vi "GISStatus_XML_Read.vi"(8 "error in (no error)":errorcluster, 11 "XML String":string="<?xml version=\"1.0\" encoding=\"utf-8\"?>\n<PrintHeadStatusXML>    \n\t<PrintManager Name=\"Print Manager\" NodeName=\"PrintManager\" Type=\"1\">        \n\t\t<PrintLineManager Name=\"Print Line Manager\" NodeName=\"PrintLineManager\" Type=\"2\">            \n\t\t\t<PrintManagerBoard Name=\"PMB-KM\" NodeName=\"PrintManagerBoard\" Type=\"3\">                \n\t\t\t\t<H Name=\"HIB1-KM1024i\" NodeName=\"HIB\" Type=\"4\" Handle=\"000001B03748C210\" HeadEnabled=\"True\" SpitEnabled=\"True\" Status=\"16\" HeaterEnabled=\"True\" TargetTemperature=\"0.00000000\" CurrentTemperature=\"23.40000000\"/>                \n\t\t\t\t<H Name=\"HIB2-KM1024i\" NodeName=\"HIB\" Type=\"4\" Handle=\"000001B03904CD00\" HeadEnabled=\"True\" SpitEnabled=\"True\" Status=\"16\" HeaterEnabled=\"True\" TargetTemperature=\"0.00000000\" CurrentTemperature=\"23.20000000\"/>                \n\t\t\t\t<H Name=\"HIB3-KM1024i\" NodeName=\"HIB\" Type=\"4\" Handle=\"000001B03AB59010\" HeadEnabled=\"True\" SpitEnabled=\"True\" Status=\"16\" HeaterEnabled=\"True\" TargetTemperature=\"0.00000000\" CurrentTemperature=\"23.40000000\"/>                \n\t\t\t\t<H Name=\"HIB4-KM1024i\" NodeName=\"HIB\" Type=\"4\" Handle=\"000001B03BFC6030\" HeadEnabled=\"True\" SpitEnabled=\"True\" Status=\"16\" HeaterEnabled=\"True\" TargetTemperature=\"0.00000000\" CurrentTemperature=\"23.20000000\"/>                \n\t\t\t\t<H Name=\"HIB5-KM1024i\" NodeName=\"HIB\" Type=\"4\" Handle=\"000001B03CF9BF40\" HeadEnabled=\"True\" SpitEnabled=\"True\" Status=\"16\" HeaterEnabled=\"True\" TargetTemperature=\"0.00000000\" CurrentTemperature=\"23.20000000\"/>                \n\t\t\t\t<H Name=\"HIB6-KM1024i\" NodeName=\"HIB\" Type=\"4\" Handle=\"000001B03DF5A440\" HeadEnabled=\"True\" SpitEnabled=\"True\" Status=\"16\" HeaterEnabled=\"True\" TargetTemperature=\"0.00000000\" CurrentTemperature=\"23.10000000\"/>            \n\t\t\t</PrintManagerBoard>        \n\t\t</PrintLineManager>    \n\t</PrintManager>\n</PrintHeadStatusXML>") -> (0 "error out":errorcluster, 2 "HeadStatus":T1[](array[typedef]), 3 "data":T2)   [LabVIEW 2022 SP3]
uses:
  Controls/SystemStatus_HT_R--cluster.ctl
  Classes/GIS Printer/Typedefs/GIS Status--Cluster.ctl
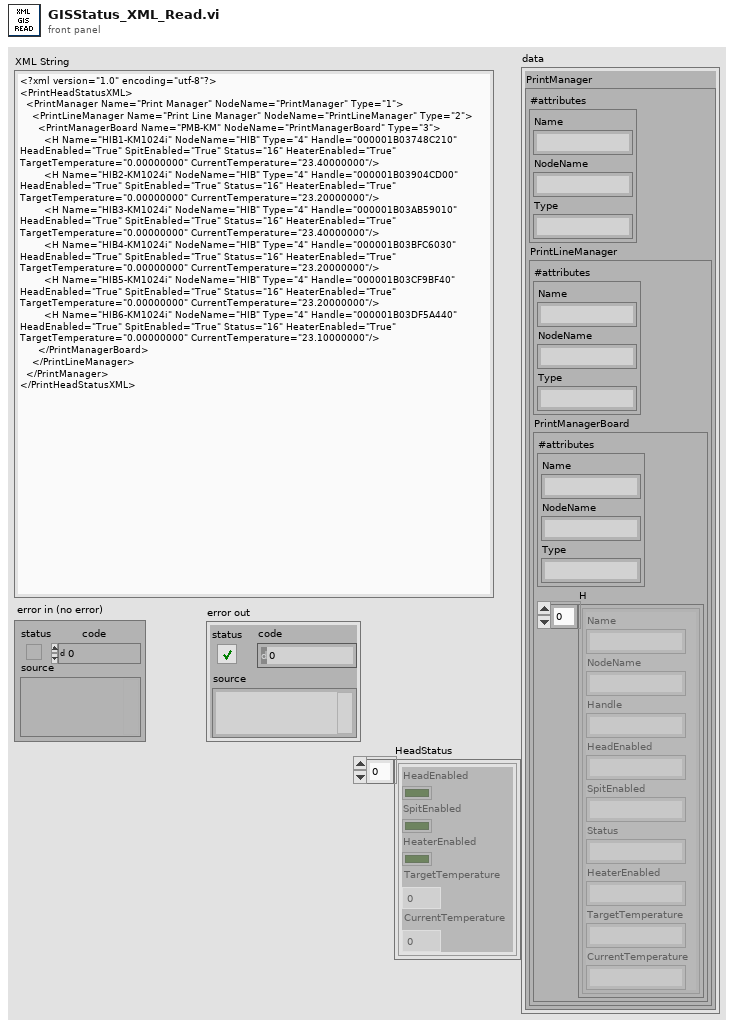
[diagram p1: front panel]
types:
  T1 = typedef "GIS Status--Cluster.ctl" = cluster{"HeadEnabled":bool, "SpitEnabled":bool, "HeaterEnabled":bool, "TargetTemperature":dbl, "CurrentTemperature":dbl}
  T2 = typedef "SystemStatus_HT_R--cluster.ctl" = cluster{"PrintManager":cluster{"#attributes":cluster{"Name":string, "NodeName":string, "Type":string}, "PrintLineManager":cluster{"#attributes":cluster{"Name":string, "NodeName":string, "Type":string}, "PrintManagerBoard":cluster{"#attributes":cluster{"Name":string, "NodeName":string, "Type":string}, "H":cluster{"Name":string, "NodeName":string, "Handle":string, "HeadEnabled":string, "SpitEnabled":string, "Status":string, "HeaterEnabled":string, "TargetTemperature":string, "CurrentTemperature":string}[]}}}}
  T3 = cluster{"PrintManager":cluster{"#attributes":cluster{"Name":string, "NodeName":string, "Type":string}, "PrintLineManager":cluster{"#attributes":cluster{"Name":string, "NodeName":string, "Type":string}, "PrintManagerBoard":cluster{"#attributes":cluster{"Name":string, "NodeName":string, "Type":string}, "H":cluster{"Name":string, "NodeName":string, "Handle":string, "HeadEnabled":string, "SpitEnabled":string, "Status":string, "HeaterEnabled":string, "TargetTemperature":string, "CurrentTemperature":string}[]}}}}
  T4 = cluster{"Name":string, "NodeName":string, "Handle":string, "HeadEnabled":string, "SpitEnabled":string, "Status":string, "HeaterEnabled":string, "TargetTemperature":string, "CurrentTemperature":string}[]
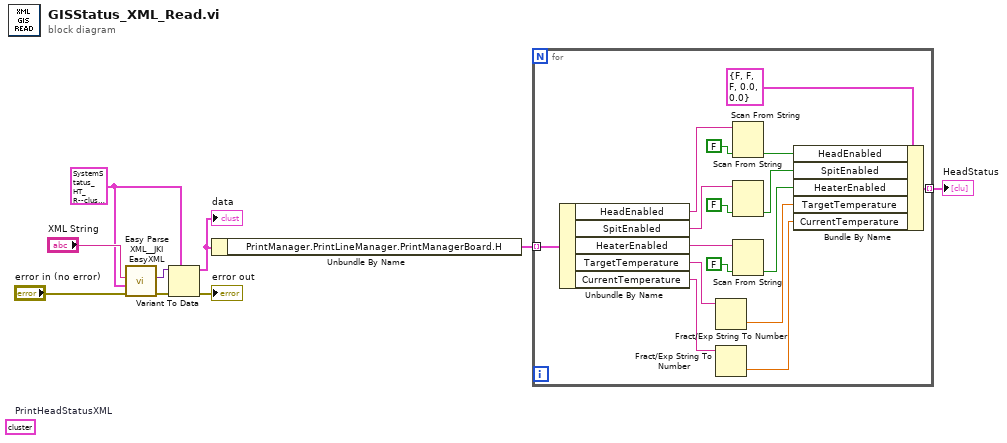
[diagram p0: block diagram]
diagram:
  w4 = T2 {"PrintManager"={"#attributes"={"Name"="Print Manager", "NodeName"="PrintManager", "Type"="1"}, "PrintLineManager"={"#attributes"={"Name"="Print Line Manager", "NodeName"="PrintLineManager", "Type"="2"}, "PrintManagerBoard"={"#attributes"={"Name"="PMB-KM", "NodeName"="PrintManagerBoard", "Type"="3"}, "H"=[]}}}} ("data 2")
  (unwired) T3 {"PrintManager"={"#attributes"={"Name"="", "NodeName"="", "Type"=""}, "PrintLineManager"={"#attributes"={"Name"="", "NodeName"="", "Type"=""}, "PrintManagerBoard"={"#attributes"={"Name"="", "NodeName"="", "Type"=""}, "H"=[]}}}}  # PrintHeadStatusXML
  n1 = call <vilib>:"Easy Parse XML__JKI EasyXML.vi"("error in (no error)"="error in (no error)", "LabVIEW Data (Type)"=w4, "XML String"="XML String") -> ("error out"=w7:errorcluster, "LabVIEW Data"=w8:variant)  [unwired: 7 in]
  n2 = Variant To Data(error in=w7, type=w4, Variant=w8) -> (data=w3:T2, error out=→"error out":errorcluster)
  "data" <- w3
  n3 = Unbundle By Name(w3) -> ("PrintManager.PrintLineManager.PrintManagerBoard.H"=w2:T4)
  n4 = for {
    tunnel: w2 -> [w25] mode=indexing
    tunnel: [w10] -> w1 mode=indexing
    n5 = Unbundle By Name(w25) -> ("HeadEnabled"=w23:string, "SpitEnabled"=w19:string, "HeaterEnabled"=w16:string, "TargetTemperature"=w14:string, "CurrentTemperature"=w13:string)
    n6 = Fract/Exp String To Number(string=w14) -> (number=w12:dbl)  [unwired: 3 in, 1 out]
    n7 = Fract/Exp String To Number(string=w13) -> (number=w11:dbl)  [unwired: 3 in, 1 out]
    n8 = Scan From String(input string=w23, default 1=FALSE) -> (output 1=w21:bool)  [unwired: 3 in, 3 out]
    n9 = Scan From String(input string=w19, default 1=FALSE) -> (output 1=w18:bool)  [unwired: 3 in, 3 out]
    n10 = Scan From String(input string=w16, default 1=FALSE) -> (output 1=w15:bool)  [unwired: 3 in, 3 out]
    n11 = Bundle By Name(cluster=T1 {"HeadEnabled"=FALSE, "SpitEnabled"=FALSE, "HeaterEnabled"=FALSE, "TargetTemperature"=0.0, "CurrentTemperature"=0.0} ("GISStatus"), "HeadEnabled"=w21, "SpitEnabled"=w18, "HeaterEnabled"=w15, "TargetTemperature"=w12, "CurrentTemperature"=w11) -> (w10:T1)
  }
  "HeadStatus" <- w1
